vi "Agilent 34420 Read Math.vi"() -> ()   [LabVIEW 2021]
doc: "This example shows how to use the math functionality of the 34420."
uses:
  <instrlib>/Agilent 34420/Public/Data/Read (Math).vi
  <instrlib>/Agilent 34420/Agilent 34420.lvlib
panel:
  in  "Maximum Time (30000 ms)":u32=30000
  out "Measurement Count":dbl
  out "Standard Deviation":dbl
  out "Average":dbl
  out "Maximum Value":dbl
  out "Minimum Value":dbl
  in  "Sample Count (1)":i32=1 format="%#.6g"
  in  "Trigger Count (1)":i32=1 format="%#.6g"
  in  "Function (0: DC Volts)":u16(ring) items=["DC Volts", "DC Voltage Ratio", "DC Voltage Difference", "2 Wire Resistance", "4 Wire Resistance", "Temperature"]
  in  "Serial Configuration":T1={"Baud Rate"=9600, "Parity"=0, "Data Bits"=8} {"Data Bits" items=["7"=7, "8"=8]; "Parity" items=["None", "Odd", "Even", "Mark", "Space"]; "Baud Rate" items=["300"=300, "600"=600, "1200"=1200, "2400"=2400, "4800"=4800, "9600"=9600]}
  in  "VISA resource name":refnum<visa-resource-name>
  # "(c) 2008-2015 National Instruments Corp.  ALL RIGHTS RESERVED."
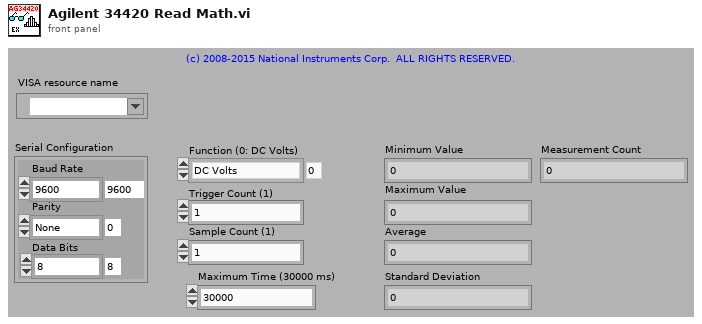
[diagram p1: front panel]
types:
  T1 = cluster{"Baud Rate":u32, "Parity":u16, "Data Bits":u16}
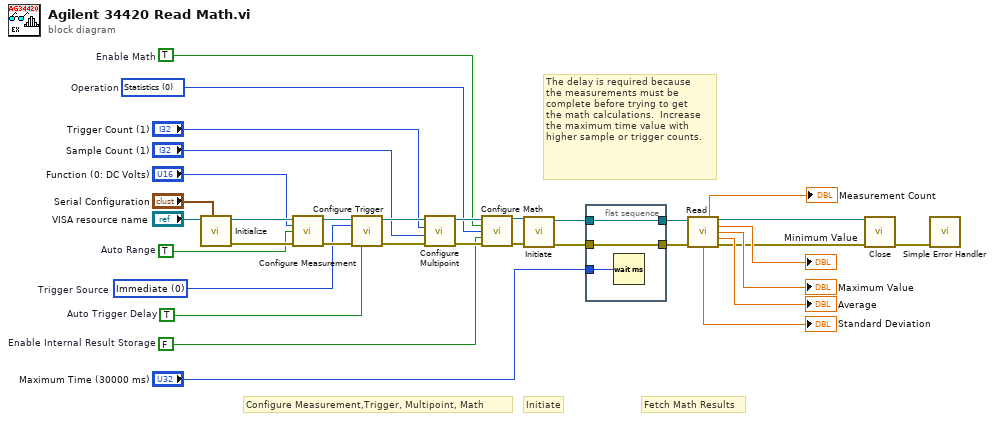
[diagram p0: block diagram]
diagram:
  w1 = TRUE  # Auto Trigger Delay
  w2 = FALSE  # Enable Internal Result Storage
  w17 = u16 0 items=["Statistics", "Scaling"]  # Operation
  w18 = TRUE  # Enable Math
  w25 = u16 0 items=["Immediate", "Software (Bus)", "External"]  # Trigger Source
  w26 = TRUE  # Auto Range
  # "The delay is required because\nthe measurements must be\ncomplete before trying to get\nthe math calculations.  Increase\nthe maximum time value with \nhigher sample or trigger counts."
  # "Fetch Math Results"
  # "Initiate"
  # "Configure Measurement,Trigger, Multipoint, Math"
  n1 = call <instrlib>:"Initialize.vi"("Serial Configuration"="Serial Configuration", "VISA resource name"="VISA resource name") -> ("error out"=w32:errorcluster, "VISA resource name out"=w33:refnum<visa-resource-name>)  [unwired: 8 in]
  n2 = call <instrlib>:"Configure Measurement.vi"("VISA resource name"=w33, "Function (0: DC Volts)"="Function (0: DC Volts)", "Auto Range (T:Enable)"=w26, "error in (no error)"=w32) -> ("VISA resource name out"=w31:refnum<visa-resource-name>, "error out"=w30:errorcluster)  [unwired: 10 in]
  n3 = call <instrlib>:"Configure Trigger.vi"("VISA resource name"=w31, "Trigger Source (0: Immediate)"=w25, "error in (no error)"=w30, "Auto Trigger Delay (T:Enable)"=w1) -> ("VISA resource name out"=w29:refnum<visa-resource-name>, "error out"=w28:errorcluster)  [unwired: 10 in]
  n4 = call <instrlib>:"Configure Multipoint.vi"("error in (no error)"=w28, "Sample Count (1)"="Sample Count (1)", "Trigger Count (1)"="Trigger Count (1)", "VISA resource name"=w29) -> ("error out"=w22:errorcluster, "VISA resource name out"=w21:refnum<visa-resource-name>)  [unwired: 6 in]
  n5 = call <instrlib>:"Configure Math.vi"("VISA resource name"=w21, "Enable Math (T: Enable)"=w18, "Operation (0: Statistics)"=w17, "Enable Internal Result Storage (T: Enable)"=w2, "error in (no error)"=w22) -> ("VISA resource name out"=w19:refnum<visa-resource-name>, "error out"=w20:errorcluster)  [unwired: 9 in]
  n6 = call <instrlib>:"Initiate.vi"("error in (no error)"=w20, "VISA resource name"=w19) -> ("error out"=w7:errorcluster, "VISA resource name out"=w9:refnum<visa-resource-name>)  [unwired: 8 in]
  n7 = flat-sequence {
    tunnel: [w37] -> w8
    tunnel: w9 -> [w37]
    tunnel: [w36] -> w6
    tunnel: w7 -> [w36]
    tunnel: "Maximum Time (30000 ms)" -> [w35]
    frame #0 {
      n8 = Wait (ms)(milliseconds to wait=w35) -> ()  [unwired: 1 out]
    }
  }
  n9 = call-poly <instrlib>:"Read.vi"("VISA resource name"=w8, "error in (no error)"=w6) -> ("Measurement Count"=→"Measurement Count":dbl, "VISA resource name out"=w4:refnum<visa-resource-name>, "Minimum Value"=→"Minimum Value":dbl, "Maximum Value"=→"Maximum Value":dbl, "Average"=→"Average":dbl, "Standard Deviation"=→"Standard Deviation":dbl, "error out"=w3:errorcluster)  [unwired: 6 in, 1 out]
  n10 = call <instrlib>:"Close.vi"("error in (no error)"=w3, "VISA resource name"=w4) -> ("error out"=w27:errorcluster)  [unwired: 9 in]
  n11 = call <vilib>:"Simple Error Handler.vi"("error in (no error)"=w27) -> ()  [unwired: 4 in, 5 out]
